vi "EIP Instance Section.vi"(8 "error in (no error)":errorcluster, 11 "Node Ptr":T4 format="%.0x") -> (0 "error out":errorcluster)   [LabVIEW 2023, in "Ethernet IP Custom Device Custom Device.lvlib"]
uses:
  Ethernet IP Custom Device Custom Device.lvlib
  <vilib>/NI VeriStand/Custom Device API/Custom Device Item Ref.ctl
  EIP Message Type.ctl
  EIP Attribute Channel Info.ctl
  EIP Attribute Direction.ctl
  Ethernet IP Global Strings.vi
  <vilib>/NI VeriStand/Custom Device API/Get Item Property (Variant).vi
  <vilib>/NI VeriStand/Custom Device API/Custom Device API.lvlib
panel:
  out "assembly info":T1
  out "message type":T3
  in  "Description":string
  in  "Header":cluster{"Section Name":string}={"Section Name"="Custom Device Item Settings"}
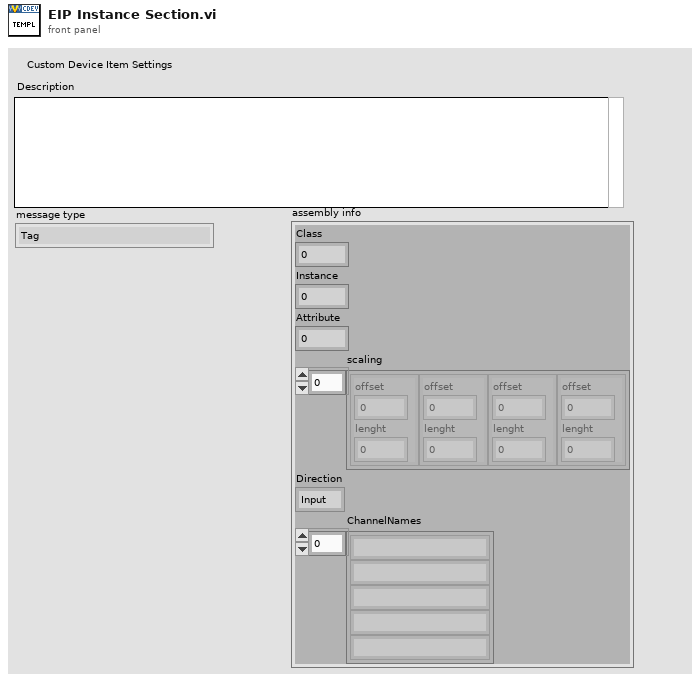
[diagram p1: front panel]
types:
  T1 = typedef "Ethernet IP Custom Device Custom Device.lvlib/EIP Attribute Channel Info.ctl" = cluster{"Class":i32, "Instance":u32, "Attribute":i32, "scaling":cluster{"offset":u32, "lenght":u32}[], "Direction":T2, "ChannelNames":string[]}
  T2 = typedef "Ethernet IP Custom Device Custom Device.lvlib/EIP Attribute Direction.ctl" = enum16{"Input", "Output"}
  T3 = typedef "Ethernet IP Custom Device Custom Device.lvlib/EIP Message Type.ctl" = enum16{"Tag", "Assembly"}
  T4 = typedef "Custom Device API.lvlib/Custom Device Item Ref.ctl" = u64
  T5 = typedef "Custom Device API.lvlib/Custom Device Commands.ctl" = enum16{"Default", "Item renamed", "Shutdown", "Dynamic button pressed"}
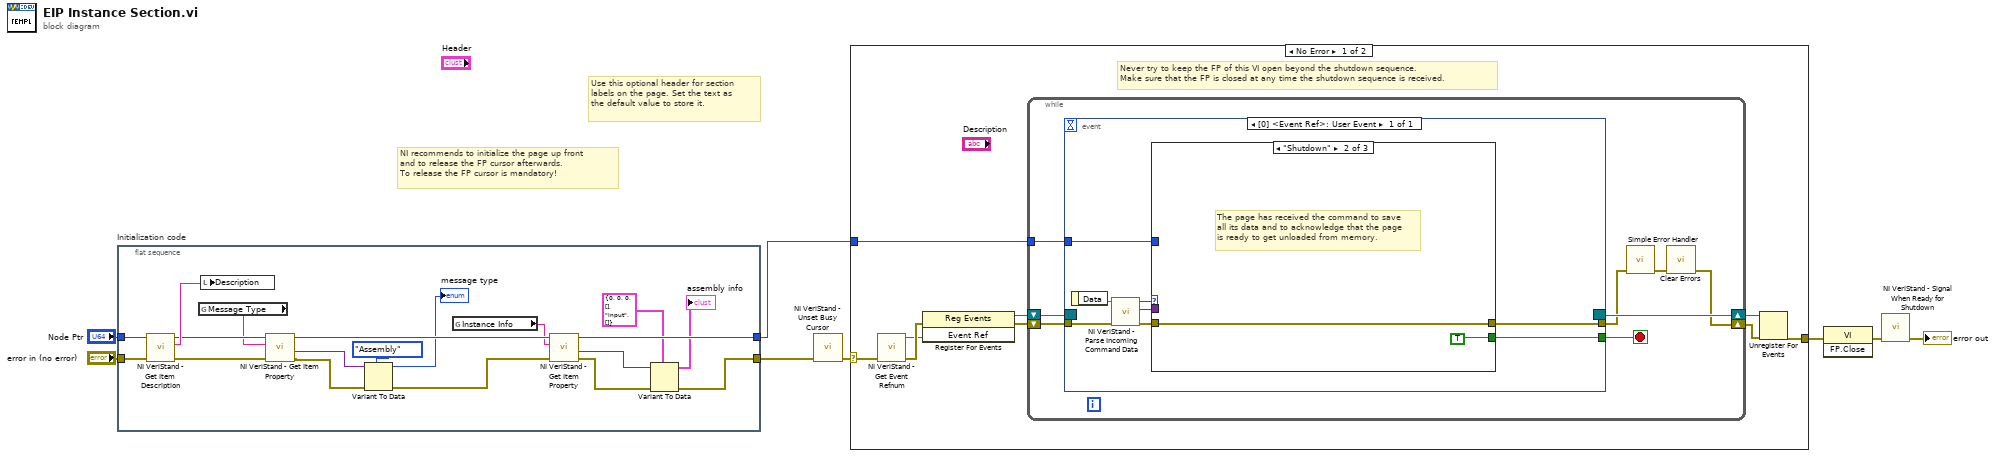
[diagram p0: block diagram]
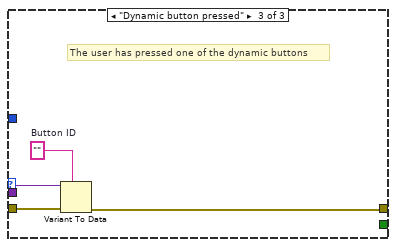
[diagram p3: hidden frame]
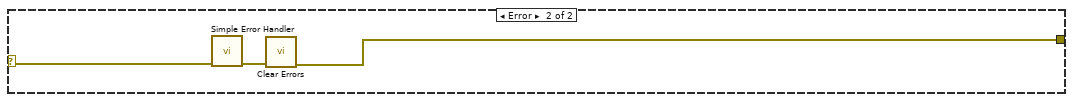
[diagram p4: hidden frame]
diagram:
  # "Use this optional header for section labels on the page. Set the text as the default value to store it."
  # "NI recommends to initialize the page up front\nand to release the FP cursor afterwards.\nTo release the FP cursor is mandatory!"
  n1 = flat-sequence "Initialization code" {
    tunnel: "error in (no error)" -> [w27]
    tunnel: "Node Ptr" -> [w26]
    tunnel: [w21] -> w2
    tunnel: [w11] -> w1
    frame #0 {
      n2 = call <vilib>:"NI VeriStand - Get Item Description.vi"("error in (no error)"=w27, "Item Ref in"=w26) -> ("error out"=w24:errorcluster, "Description"=w25:string, "Item Ref out"=w22:T4)  [unwired: 7 out]
      n3 = global read "Ethernet IP Global Strings.vi" "Message Type"() -> (w20:string)
      n4 = local write "Description"(w25) -> ()
      n5 = call-poly <vilib>:"NI VeriStand - Get Item Property.vi"("error in (no error)"=w24, "Property Name"=w20, "Item Ref in"=w22) -> ("error out"=w18:errorcluster, "Value"=w19:variant, "Item Ref out"=w23:T4)  [unwired: 5 in, 1 out]
      n6 = Variant To Data(error in=w18, type=EIP_Message_Type."Assembly" ("Message Type"), Variant=w19) -> (data=→"message type":T3, error out=w15:errorcluster)
      n7 = global read "Ethernet IP Global Strings.vi" "Instance Info"() -> (w14:string)
      n8 = call-poly <vilib>:"NI VeriStand - Get Item Property.vi"("error in (no error)"=w15, "Property Name"=w14, "Item Ref in"=w23) -> ("error out"=w13:errorcluster, "Value"=w12:variant, "Item Ref out"=w21:T4)  [unwired: 5 in, 1 out]
      n9 = Variant To Data(error in=w13, type=T1 {"Class"=0, "Instance"=0, "Attribute"=0, "scaling"=[], "Direction"=enum."Input", "ChannelNames"=[]} ("Attribute Info"), Variant=w12) -> (data=→"assembly info":T1, error out=w11:errorcluster)
    }
  }
  n10 = call <vilib>:"NI VeriStand - Unset Busy Cursor.vi"("error in (no error)"=w1) -> ("error out"=w4:errorcluster)  [unwired: 10 out]
  n11 = case shown="No Error" w4 {
    selector: w4 -> [w28 w62]
    tunnel: [w33 w60] -> w8
    tunnel: w2 -> [w29 _]
    frame No Error {
      # "Never try to keep the FP of this VI open beyond the shutdown sequence.\nMake sure that the FP is closed at any time the shutdown sequence is received."
      n12 = call <vilib>:"NI VeriStand - Get Event Refnum.vi"("error in (no error)"=w28) -> ("error out"=w36:errorcluster, "Event Ref"=w32:refnum<user-event>)  [unwired: 9 out]
      n13 = register-events(error in=w36, w32) -> (reference out=w30:refnum<event-registration>, error out=w31:errorcluster)  [unwired: 1 in]
      n14 = while {
        tunnel: w29 -> [w40]
        shift-right: [w37] -> w34
        shift-left: w31 -> [w43]
        shift-right: [w44] -> w35
        shift-left: w30 -> [w42]
        stop <- w41 stop-if-true
        n15 = event shown="[0] <Event Ref>: User Event" {
          selector: w42 -> [_]
          dyn-events: [_] -> w44
          timeout: _ -> [_]
          tunnel: w43 -> [w52]
          tunnel: [w48] -> w41
          tunnel: [w47] -> w39
          tunnel: w40 -> [w46]
          event User Event {
            n16 = event-data() -> ("Data"=w51:string)  [unwired: 1 out]
            n17 = call <vilib>:"NI VeriStand - Parse Incoming Command Data.vi"("error in (no error)"=w52, "Incoming data"=w51) -> ("error out"=w50:errorcluster, "Outgoing data"=w45:variant, "Action"=w49:T5)  [unwired: 7 out]
            n18 = case shown="\"Shutdown\"" w49 {
              tunnel: w50 -> [w53 w54 w59]
              tunnel: [_ TRUE _] -> w48
              tunnel: [w53 w54 w56] -> w47
              tunnel: w46 -> [_ _ _]
              tunnel: w45 -> [_ _ w58]
              frame "Default", Default {
              }
              frame "Shutdown" {
                # "The page has received the command to save all its data and to acknowledge that the page is ready to get unloaded from memory."
              }
              frame "Dynamic button pressed" {
                w57 = ""  # Button ID
                # "The user has pressed one of the dynamic buttons"
                n19 = Variant To Data(error in=w59, type=w57, Variant=w58) -> (error out=w56:errorcluster)  [unwired: 1 out]
              }
            }
          }
        }
        n20 = call <vilib>:"Simple Error Handler.vi"("error in (no error)"=w39) -> ("error out"=w38:errorcluster)  [unwired: 1 in, 7 out]
        n21 = call <vilib>:"Clear Errors.vi"("error in (no error)"=w38) -> ("error out"=w37:errorcluster)  [unwired: 1 in, 5 out]
      }
      n22 = Unregister For Events(event registration refnum=w35, error in=w34) -> (error out=w33:errorcluster)
    }
    frame Error {
      n23 = call <vilib>:"Simple Error Handler.vi"("error in (no error)"=w62) -> ("error out"=w61:errorcluster)  [unwired: 1 in, 7 out]
      n24 = call <vilib>:"Clear Errors.vi"("error in (no error)"=w61) -> ("error out"=w60:errorcluster)  [unwired: 1 in, 5 out]
    }
  }
  n25 = invoke class="VI" method="FP.Close"(error in=w8) -> (error out=w7:errorcluster)  [unwired: 2 in, 2 out]
  n26 = call <vilib>:"NI VeriStand - Signal When Ready for Shutdown.vi"("error in (no error)"=w7) -> ("error out"=→"error out":errorcluster)  [unwired: 10 out]
